vi "Send Data.vi"(8 "error in":errorcluster, 10 "Data":refnum<class "Data.lvclass">, 11 "DAQ Device in":refnum<class "DAQ Device.lvclass">) -> (0 "error out":errorcluster, 3 "DAQ Device out":refnum<class "DAQ Device.lvclass">)   [LabVIEW 2014, in "DAQ Device.lvclass"]
uses:
  DAQ Device.lvclass
  Data/Data.lvclass
  <vilib>/ActorFramework/Actor/Actor.lvclass/Actor.ctl
  DAQ Device.lvclass/DAQ Device.ctl
  Messages/Send Data Msg.lvclass/Send Data Msg.ctl
  <vilib>/ActorFramework/Message Enqueuer/Message Enqueuer.lvclass/Message Enqueuer.ctl
  <vilib>/ActorFramework/Message Priority Queue/Priority Enqueue.vi
  <vilib>/ActorFramework/Actor/Actor.lvclass
  <vilib>/ActorFramework/Message Enqueuer/Message Enqueuer.lvclass
  Messages/Send Data Msg.lvclass
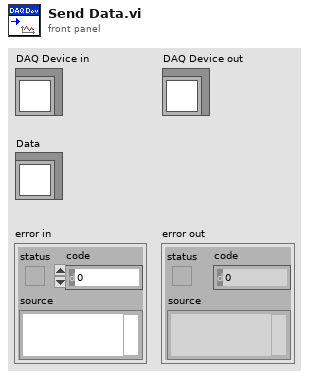
[diagram p1: front panel]
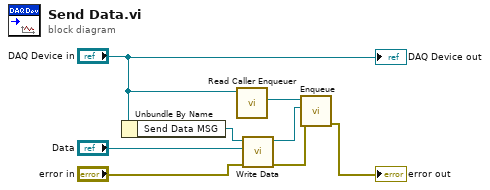
[diagram p0: block diagram]
diagram:
  n1 = Unbundle By Name("DAQ Device in") -> ("Send Data MSG"=w5:refnum<class "Send Data Msg.lvclass">)
  n2 = call <vilib>:"Read Caller Enqueuer.vi"("Actor"="DAQ Device in") -> ("Caller Enqueuer"=w6:refnum<class "Message Enqueuer.lvclass">)  [unwired: 10 in]
  n3 = call "Write Data.vi"("error in"="error in", "Data"="Data", "Send Data Msg in"=w5) -> ("error out"=w3:errorcluster, "Send Data Msg out"=w4:refnum<class "Send Data Msg.lvclass">)  [unwired: 7 in]
  n4 = call <vilib>:"Enqueue.vi"("error in (no error)"=w3, "Message"=w4, "Message Enqueuer in"=w6) -> ("error out"=→"error out":errorcluster)  [unwired: 7 in, 1 out]
  "DAQ Device out" <- "DAQ Device in"
